vi "Launcher.vi"   [LabVIEW 2019]
uses:
  Modules/Core/Core.lvclass
  C:/Program Files (x86)/National Instruments/LabVIEW 2019/vi.lib/ActorFramework/Actor/Actor.lvclass
  <vilib>/ActorFramework/Actor/Actor.lvclass
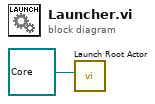
[diagram p0: block diagram]
diagram:
  n1 = call <vilib>:"Launch Root Actor.vi"("Actor"=refnum<class "Core.lvclass"> refnum ("Core.lvlib:Core.lvclass")) -> ()  [unwired: 9 in, 2 out]
